vi "Zaber Intermediate - Read Input from User and Display Responses.vi"() -> ()   [LabVIEW 2020]
doc: "By default, this example behaves the same as the previous one, but now it asks the user how many moves to make, how big each move should be, and which device to use. It also displays all the responses from the device.\nThe block diagram shows how to read input from controls and display output in indicators. It also shows how to build a request cluster using the Bundle function and then change it using the Bundle By Name function. It uses a self test to make sure that the device is connected before we start sending move commands. In addition to the error and COM port wires, we now have a Responses wire flowing along the bottom of\nthe diagram. We wire the responses indicator inside the loop so that the response list will get updated after each command finishes."
uses:
  Public/Utility/Response.ctl
  ZaberTSeries.lvlib
panel:
  out "Responses":T1[](array[typedef]) {"Command" items=["Constant Speed Tracking"=8, "Echo"=55, "Error"=255, "Home"=1, "Limit Active"=9, "Manual Move Tracking"=10, "Move Absolute"=20, "Move at Constant Speed"=22, "Move Relative"=21, "Renumber"=2, "Restore Settings"=36, "Stop"=23]}
  in  "Move Size":i32=10000
  in  "Device Number":u8=1
  in  "Move Count":i32=5
  in  "VISA resource name":refnum<visa-resource-name>
  # "By default, this behaves the same as the previous examples,\nbut now it asks  the user how many moves to make, how big\neach move should be, and which device to use.  It also displays\nall the responses from the device.\nType Ctrl-E to see how the block diagram is wired."
  # "Don't use device 0."
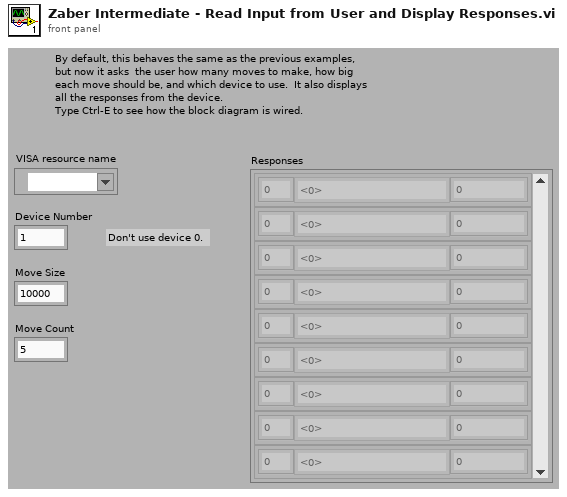
[diagram p1: front panel]
types:
  T1 = typedef "ZaberTSeries.lvlib/Response.ctl" = cluster{"Device Number":u8, "Command":u8, "Data":i32}
  T2 = cluster{"Device Number":u8, "Command":u8, "Data":i32, "Response Count":i32}
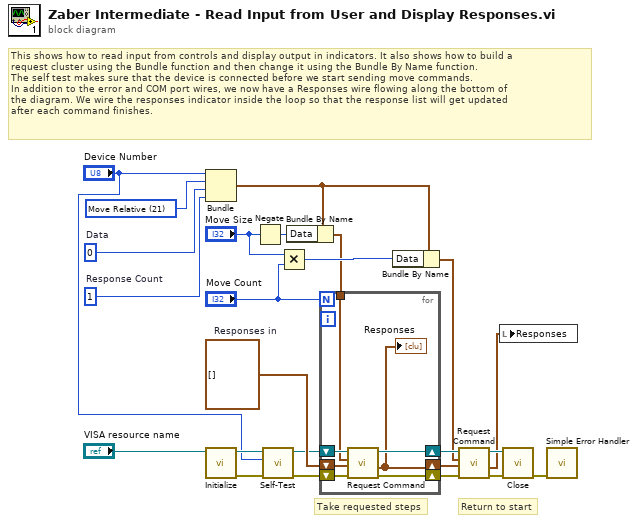
[diagram p0: block diagram]
diagram:
  w9 = 0  # Data
  w13 = 1  # Response Count
  w14 = u8 21 items=["Echo"=55, "Home"=1, "Move Absolute"=20, "Move Relative"=21, "Move at Constant Speed"=22, "Renumber"=2, "Restore Settings"=36, "Stop"=23] ("Command")
  w17 = T1[] []  # Responses in
  # "This shows how to read input from controls and display output in indicators. It also shows how to build a \nrequest cluster using the Bundle function and then change it using the Bundle By Name function.\nThe self test makes sure that the device is connected before we start sending move commands.\nIn addition to the error and COM port wires, we now have a Responses wire flowing along the bottom of\nthe diagram. We wire the responses indicator inside the loop so that the response list will get updated \nafter each command finishes."
  # "Return to start"
  # "Take requested steps"
  n1 = Bundle("Device Number"="Device Number", "Command"=w14, "Data"=w9, "Response Count"=w13) -> (w8:T2)  [unwired: 1 in]
  n2 = call "Initialize.vi"("VISA resource name"="VISA resource name") -> ("error out"=w5:errorcluster, "VISA resource name out"=w4:refnum<visa-resource-name>)  [unwired: 8 in, 1 out]
  n3 = Negate(x="Move Size") -> (-x=w6:i32)
  n4 = call "Self-Test.vi"("error in (no error)"=w5, "Device Number"="Device Number", "VISA resource name"=w4) -> ("error out"=w1:errorcluster, "VISA resource name out"=w2:refnum<visa-resource-name>)  [unwired: 5 in, 2 out]
  n5 = Multiply(x="Move Size", y="Move Count") -> (x*y=w11:i32)
  n6 = Bundle By Name(cluster=w8, "Data"=w6) -> (w7:T2)
  n7 = for {
    N: "Move Count" -> [_]
    shift-right: [w26] -> w15
    shift-left: w17 -> [w27]
    shift-right: [w28] -> w19
    shift-left: w1 -> [w31]
    tunnel: w7 -> [w25]
    shift-right: [w29] -> w20
    shift-left: w2 -> [w30]
    n8 = call "Request Command.vi"("error in (no error)"=w31, "Responses in"=w27, "Request"=w25, "VISA resource name"=w30) -> ("error out"=w28:errorcluster, "Responses out"=w26:T1[], "VISA resource name out"=w29:refnum<visa-resource-name>)  [unwired: 4 in, 1 out]
    "Responses" <- w26
  }
  n9 = Bundle By Name(cluster=w8, "Data"=w11) -> (w18:T2)
  n10 = call "Request Command.vi"("error in (no error)"=w19, "Responses in"=w15, "Request"=w18, "VISA resource name"=w20) -> ("error out"=w22:errorcluster, "Responses out"=w16:T1[], "VISA resource name out"=w23:refnum<visa-resource-name>)  [unwired: 4 in, 1 out]
  n11 = local write "Responses"(w16) -> ()
  n12 = call "Close.vi"("error in (no error)"=w22, "VISA resource name"=w23) -> ("error out"=w24:errorcluster)  [unwired: 8 in, 1 out]
  n13 = call <vilib>:"Simple Error Handler.vi"("error in (no error)"=w24) -> ()  [unwired: 4 in, 5 out]
